vi "sta_make linear equation (SubVI).vi"(0 "test result":dbl[](array[numeric]), 5 "factors":dbl[][](array[numeric]), 7 "name":string[](array[string]), 11 "에러 입력(에러 없음)":errorcluster) -> (4 "참조 번호 출력":refnum<k35>, 6 "sumary":string, 8 "pValue sort":dbl[](array[numeric]), 10 "name sort":string[](array[string]), 14 "coef":dbl[](array[numeric]), 15 "에러 출력":errorcluster)   [LabVIEW 2018]
uses:
  PythonConfigGlobal.vi
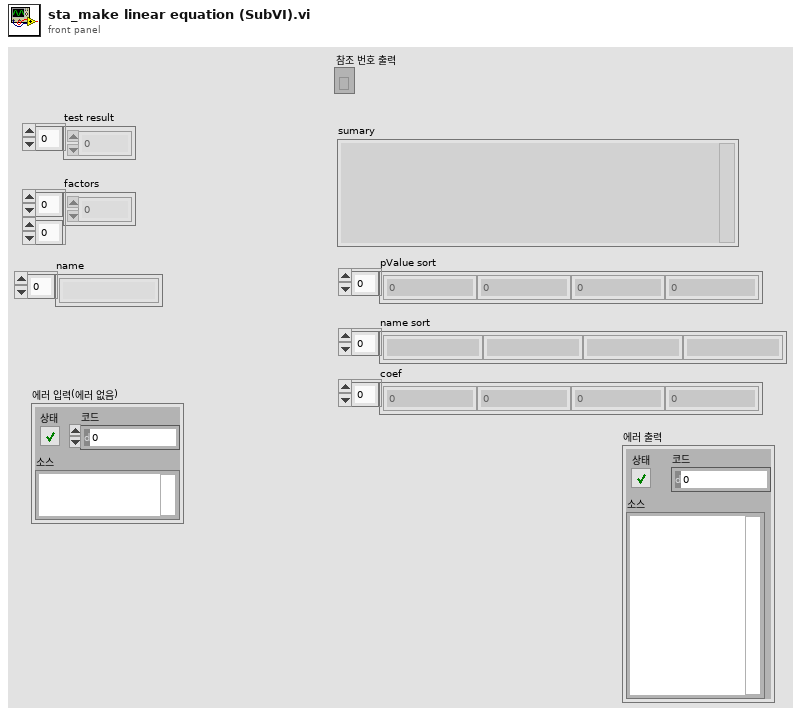
[diagram p1: front panel]
types:
  T1 = cluster{"sumary":string, "Pvalue":dbl[], "coef":dbl[]}
  T2 = cluster{"session out":refnum<k35>, "appended path":path}
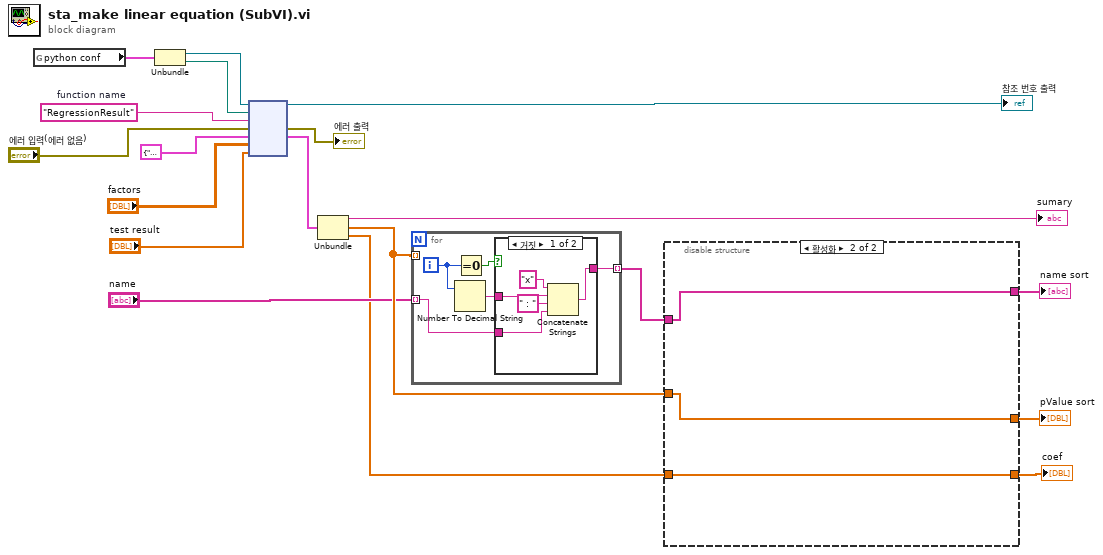
[diagram p0: block diagram]
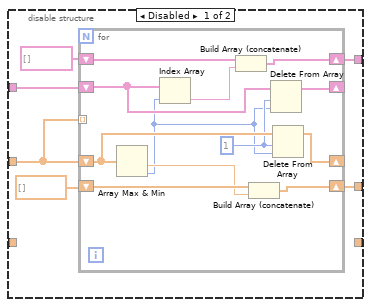
[diagram p2: hidden frame]
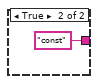
[diagram p3: hidden frame]
diagram:
  w9 = "RegressionResult"  # function name
  n1 = global read "PythonConfigGlobal.vi" "python conf"() -> (w4:T2)
  n2 = Unbundle(w4) -> ("session out"=w8:refnum<k35>, "appended path"=w7:path)
  n3 = node(w8, w7, w9, "에러 입력(에러 없음)", T1 {"sumary"="", "Pvalue"=[], "coef"=[]}, "factors", "test result") -> (→"참조 번호 출력":refnum<k35>, →"에러 출력":errorcluster, w14:T1)  [unwired: 2 in, 2 out]
  n4 = Unbundle(w14) -> ("sumary"=→"sumary":string, "Pvalue"=w19:dbl[], "coef"=w1:dbl[])
  n5 = for {
    tunnel: w19 -> [_] mode=indexing
    tunnel: [w21] -> w16 mode=indexing
    tunnel: "name" -> [w20] mode=indexing
    i -> [w23]
    n6 = Number To Decimal String(number=w23) -> (decimal integer string=w22:string)  [unwired: 1 in]
    n7 = Equal To 0?(x=w23) -> (x = 0?=w24:bool)
    n8 = case shown="거짓" w24 {
      tunnel: [w27 "const"] -> w21
      tunnel: w22 -> [w28 _]
      tunnel: w20 -> [w25 _]
      frame False {
        n9 = Concatenate Strings("x" ("문자열"), w28, " : " ("문자열"), w25) -> (w27:string)
      }
      frame True {
      }
    }
  }
  n10 = disable-structure shown="활성화" {
    disable-tunnel: w19 -> [w36 w50]
    disable-tunnel: [w35 w50] -> w18
    disable-tunnel: [w34 w51] -> w17
    disable-tunnel: w16 -> [w33 w51]
    disable-tunnel: [_ w49] -> w2
    disable-tunnel: w1 -> [_ w49]
    frame Disabled {
      n11 = for {
        shift-right: [w46] -> w35
        shift-left: dbl[] [] -> [w48]
        shift-right: [w43] -> w34
        shift-left: string[] [] -> [w44]
        shift-right: [w39] -> _
        shift-left: w33 -> [w42]
        shift-right: [w38] -> _
        shift-left: w36 -> [w41]
        tunnel: w36 -> [_] mode=indexing
        w40 = 1 ("길이")
        n12 = Array Max & Min(array=w41) -> (min value=w47:dbl, min index (indices)=w37:i32)  [unwired: 2 out]
        n13 = Index Array(array=w42, index=w37) -> (element=w45:string)
        n14 = Build Array (concatenate)(w44, w45) -> (w43:string[])
        n15 = Build Array (concatenate)(w48, w47) -> (w46:dbl[])
        n16 = Delete From Array(array=w42, length=w40, index=w37) -> (array with subset deleted=w39:string[])  [unwired: 1 out]
        n17 = Delete From Array(array=w41, length=w40, index=w37) -> (array with subset deleted=w38:dbl[])  [unwired: 1 out]
      }
    }
    frame Enabled {
    }
  }
  "name sort" <- w17
  "pValue sort" <- w18
  "coef" <- w2
